vi "SVPO Analog Tacho Process (1 Ch DBL WDT) with IC.vi"(0 "analog tacho signal":waveform(dbl)={"t0"=timestamp(0 s since 1904-01-01), "dt"=0.0, "Y"=[]}, 1 "initial conditions":T1, 2 "reset? (F)":bool, 7 "threshold":dbl format="%.2f", 9 "pulse/revolution (1)":i32=1, 11 "hysteresis (0)":dbl format="%.2f", 12 "pulse width (2)":i32=2, 13 "slope (Rising)":u16(ring) items=["Rising", "Falling"]) -> (3 "final conditions":T1, 4 "speed position info":T2, 6 "current speed [RPM]":dbl)   [LabVIEW 2017, in "SoundVib_TachProcess.lvlib"]
doc: "Locates tachometer pulse positions in analog tachometer signals using the number of generated pulses per revolution, the pulse width, and the arrival edge of the tachometer pulse. Use this VI on embedded targets that have limited computational resources. Wire data to the <B>analog tacho signal</B> input to determine the polymorphic instance to use or manually select the instance."
uses:
  <vilib>/addons/Sound and Vibration/Order Analysis/Tach Process/SoundVib_TachProcess.lvlib
  <vilib>/addons/Sound and Vibration/Order Analysis/Misc/OAT Position Info.ctl
  <vilib>/addons/_NISVFA/_Shared subVIs/Controls/svc_Analog Tacho State.ctl
  <vilib>/addons/Sound and Vibration/Order Analysis/Tach Process/SubVIs/oa_Convert Pulse Positions to Speed (No State).vi
  <vilib>/addons/Sound and Vibration/Order Analysis/Tach Process/SubVIs/sv_Edge Detection (1 Tach) with IC.vi
  <vilib>/addons/Sound and Vibration/Order Analysis/Tach Process/SubVIs/oa_Analog Tacho Hysteresis(1 Channel) with IC.vi
  <vilib>/addons/_NISVFA/_Shared subVIs/Common/SV Buffer Array (No State) (DBL).vi
  <vilib>/addons/Sound and Vibration/Order Analysis/Tach Process/SubVIs/OAT Cross Point Detection.vi
  <vilib>/addons/_NISVFA/_Shared subVIs/Common/svc_Get Array Subset (Index).vi
  <vilib>/Analysis/8numeric.llb/Threshold Detector.vi
  <vilib>/addons/_NISVFA/_Shared subVIs/Common/svc_Coerce Index and Length.vi
  <vilib>/addons/_NISVFA/_Shared subVIs/Common/svc_Conditional Merge Error.vi
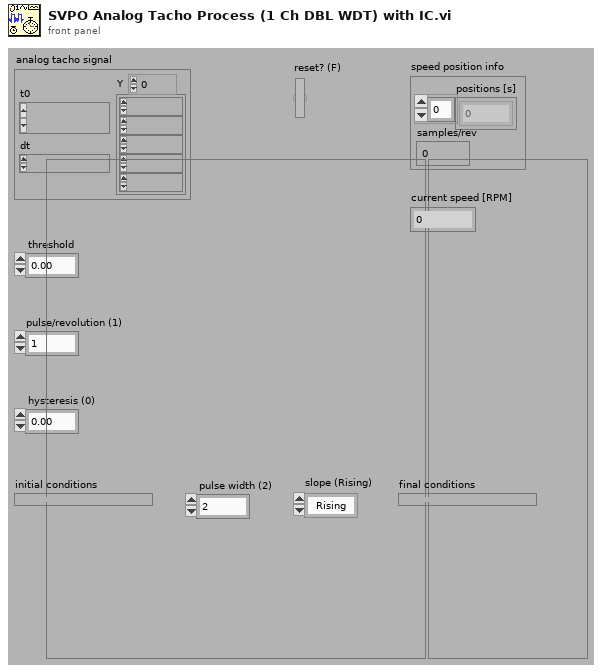
[diagram p1: front panel]
types:
  T1 = typedef "svc_Analog Tacho State.ctl" = cluster{"hysteresis state":dbl, "edge detection state":cluster{"x[n]":dbl[], "size":dbl}, "pulse to speed state":cluster{"pulse positions":dbl[], "elapsed time":dbl}}
  T2 = typedef "OAT Position Info.ctl" = cluster{"positions [s]":dbl[], "samples/rev":dbl}
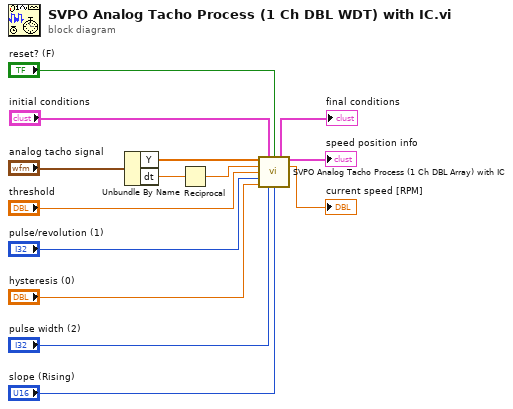
[diagram p0: block diagram]
diagram:
  n1 = Unbundle By Name("analog tacho signal") -> ("Y"=w13:dbl[], "dt"=w12:dbl)
  n2 = Reciprocal(x=w12) -> (1/x=w11:dbl)
  n3 = call <vilib>:"SVPO Analog Tacho Process (1 Ch DBL Array) with IC.vi"("analog tacho signal"=w13, "initial conditions"="initial conditions", "reset? (F)"="reset? (F)", "sampling rate [Hz]"=w11, "threshold"="threshold", "pulse/revolution (1)"="pulse/revolution (1)", "hysteresis (0)"="hysteresis (0)", "pulse width (2)"="pulse width (2)", "slope (Rising)"="slope (Rising)") -> ("final conditions"=→"final conditions":T1, "speed position info"=→"speed position info":T2, "current speed [RPM]"=→"current speed [RPM]":dbl)  [unwired: 4 in]
